vi "Draw initial figur.vi"(2 "Angle(deg)":dbl, 3 "Distance":dbl) -> (0 "Y":dbl, 1 "x":dbl)   [LabVIEW 2021]
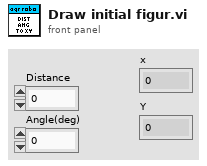
[diagram p1: front panel]
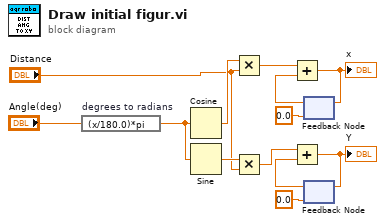
[diagram p0: block diagram]
diagram:
  n1 = expression code="(x/180.0)*pi" "degrees to radians"("Angle(deg)") -> (w9:dbl)
  n2 = Cosine(x=w9) -> (cos(x)=w11:dbl)
  n3 = Sine(x=w9) -> (sin(x)=w10:dbl)
  n4 = Multiply(x=w11, y="Distance") -> (x*y=w13:dbl)
  n5 = Multiply(x=w10, y="Distance") -> (x*y=w12:dbl)
  n6 = feedback #1(0.0) -> (w2:dbl)
  n7 = Add(x=w13, y=w2) -> (x+y=w3:dbl)
  "x" <- w3
  n8 = feedback-in #1(w3) -> ()
  n9 = feedback #2(0.0) -> (w6:dbl)
  n10 = Add(x=w12, y=w6) -> (x+y=w7:dbl)
  "Y" <- w7
  n11 = feedback-in #2(w7) -> ()
